vi "myRIO-1900 Quadrotor Motor MPU6050 FPGA.vi"() -> ()   [LabVIEW 2013]
uses:
  <vilib>/Platform/TimedLoop/XDataNode/timing_clust.ctl
  <vilib>/Platform/TimedLoop/XDataNode/nitl_modes.ctl
  <vilib>/Platform/TimedLoop/XDataNode/wakeup.ctl
  <vilib>/IEDriver/SPIandI2C/FPGA/Private/Initialize Port (I2C).vi
  <vilib>/IEDriver/SPIandI2C/FPGA/Private/IP Port (I2C).vi
  <vilib>/rvi/DataTransferAndStorage/Container/Common/niFpgaContainerGetUniqueNameForEmu.vi
  <vilib>/rvi/DataTransferAndStorage/Container/Common/niFpgaContainerSetEmuInfo.vi
  <vilib>/rvi/eio/common/nirviEmuReportErrorAndStop.vi
  <vilib>/rvi/Emulation/niFpgaSctlEmulationGetInTimedLoop.vi
  <vilib>/rvi/Emulation/niFpgaEmulationReportErrorSimple.vi
  <vilib>/rvi/Emulation/niFpgaGetClockAttributes.vi
  <vilib>/rvi/Emulation/niFpgaCriticalErrorInLSC.vi
  <vilib>/rvi/DataTransferAndStorage/Container/Common/niFpgaContainerExecOnDevCompGetState.vi
  <vilib>/rvi/FIFO/Fifo_Resource/nirvififoEmulationReadFpgaImpl.vi
  <vilib>/rvi/interface/RandomDataEmulation/nirviRandomDataFPGAFIFO.vi
  <vilib>/rvi/interface/RandomDataEmulation/niFpgaRandomDataHandleErrors.vi
  <vilib>/rvi/Memory/Memory_Emulation/nirvimemoryFastEmulationFpgaImpl.vi
  <instcachedir>/0/nirvimemoryFastEmulationFpgaImpl_5FBAB50466BC4C939F684F8805638BFC.lvgen/nirvimemoryFastEmulationFpgaImpl_5FBAB50466BC4C939F684F8805638BFC_005.vi
  <vilib>/rvi/Memory/Memory_Emulation/niFpgaMemoryEmulationCacheClearOnFirstRun.vi
  <vilib>/rvi/Memory/Memory_Emulation/nirvimemoryEmulationManagerCache_MakeExclusive.vi
  <vilib>/rvi/Memory/Memory_Emulation/niFpgaMemoryEmulationValidateCache.vi
  <vilib>/rvi/Memory/Memory_Emulation/nirvimemoryEmulationManagerCache_ReleaseExclusive.vi
  <vilib>/rvi/Memory/Memory_Emulation/nirvimemoryEmulationManagerCache_InsertValue.vi
  <vilib>/Utility/error.llb/Clear Errors.vi
  <vilib>/rvi/Memory/Memory_Emulation/nirvimemoryEmulationManagerCache_GetValue.vi
  <vilib>/rvi/Emulation/niFpgaProcessEmulError.vi
  <vilib>/rvi/eio/common/nirviEmuTemplateMethod_errors.vi
  <vilib>/IEDriver/SPIandI2C/FPGA/Private/Configure Port (I2C).vi
  <vilib>/IEDriver/SPIandI2C/FPGA/Private/Arm Port (I2C).vi
  <vilib>/IEDriver/SPIandI2C/FPGA/Private/Read Port (I2C).vi
  <vilib>/IEDriver/SPIandI2C/FPGA/Private/Write Port (I2C).vi
  <vilib>/rvi/FIFO/Fifo_Resource/nirvififoEmulationWriteFpgaImpl.vi
  <vilib>/rvi/Memory/Memory_Emulation/nirvimemoryEmulationManagerCache_SetValue.vi
  <vilib>/rvi/Emulation/niFpgaSctlEmulationResourceMgr.vi
  <vilib>/Platform/TimedLoop/XDataNode/XDataNode.xnode
  <vilib>/rvi/LocalResourceManager/LocalResourceManager.xnode
  <vilib>/rvi/DataTransferAndStorage/Container/XNode/niFpgaContainer.xnode
  <vilib>/rvi/FIFO/Fifo_Resource/niFpgaFifoEmulationRefIn.vi
  <vilib>/rvi/Memory/Memory_Emulation/niFpgaMemoryEmulationRefIn.vi
  <vilib>/eio/EIOMethodNode/EIOMethodNode.xnode
  <vilib>/Platform/TimedLoop/XDataNode/XDNodeRunTimeDep.lvlib
  <vilib>/IEDriver/SPIandI2C/FPGA/Library/IP SPI&I2C.lvlib
panel:
  in  "DataAva":bool
  out "GYR_Z":i16
  out "GYR_Y":i16
  out "GYR_X":i16
  out "TEMP":i16
  out "ACC_Z":i16
  out "ACC_Y":i16
  out "ACC_X":i16
  in  "SampleRate_Divider":u32=20000
  in  "WriteData":u8 format="0x%x"
  out "ReadData":u8 format="0x%x"
  in  "CMDParameters":T1
  in  "IICParameters":T2={"Address Type (7-bit)"=enum."7-bit", "IICSlaveAddress"=25, "I2C Parameters"={"Clock Divider"=0}} {"IICSlaveAddress" format="0x%x"}
  in  "ProtocolControl":T3(ring)
  in  "FeedDog":bool
  in  "CounterMAX":u32
  in  "PWM1":u16
  in  "PWM2":u16
  in  "PWM0":u16
  in  "PWM3":u16
  in  "MotorEn":bool
  in  "PWMOutputEN":bool
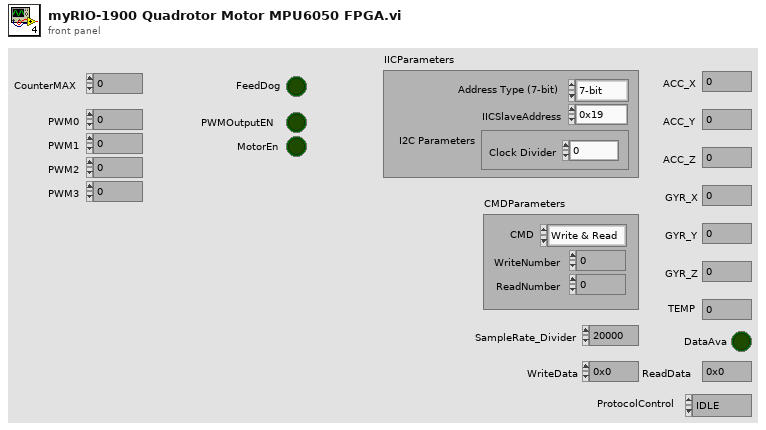
[diagram p1: front panel]
types:
  T1 = cluster{"WriteNumber":u8, "ReadNumber":u8, "CMD":enum8{"Write & Read", "Write", "Read"}}
  T2 = cluster{"Address Type (7-bit)":enum16{"7-bit", "10-bit"}, "IICSlaveAddress":u16, "I2C Parameters":cluster{"Clock Divider":u32}}
  T3 = enum8{"IDLE", "SetIDLE", "Config", "Arm", "Read", "Write", "AutoRead"}
  T4 = cluster{"MPU6050FIFO":refnum<k21>, "MPU6050FIFOAvailable":refnum<k21>}
  T5 = cluster{"PWM0":refnum<k21>, "PWM1":refnum<k21>, "PWM2":refnum<k21>, "PWM3":refnum<k21>}
  T6 = typedef "IP SPI&I2C.lvlib/Private Data (I2C).ctl" = cluster{"Arm Trigger":refnum<k21>, "API to IP Data":refnum<k21>, "IP to API Data":refnum<k21>, "Configuration Register":refnum<k21>, "Configuration Lock":refnum<k21>}
  T7 = typedef "XDNodeRunTimeDep.lvlib/timing_clust.ctl" = cluster{"Expected End [f-1]":u64, "Actual End [f-1]":u64, "Finished Late? [f-1]":bool, "Expected End [i-1]":u64, "Actual End [i-1]":u64, "Finished Late? [i-1]":bool, "Expected Start [i]":u64, "Actual Start [i]":u64, "Expected Start [f]":u64, "Actual Start [f]":u64, "Source Name":string, "Structure Name":string, "Period":i64, "Deadline":i64, "Offset":i64, "Start":i64, "Priority":i32, "Timeout":i32, "Mode":T8, "Wakeup Reason":T9, "Error":errorcluster, "Source Type":string, "Secondary Source Type":string, "Global End Time":u64, "Global Start Time":u64, "Frame Duration":u64, "Iteration Duration":u64, "Assigned CPU":i32, "I/O Scan Engine Mode":u32}
  T8 = typedef "XDNodeRunTimeDep.lvlib/nitl_modes.ctl" = enum32{"No Change", "Process missed periods, maintain original phase", "Discard missed periods, maintain original phase", "Process missed periods, ignore original phase", "Discard missed periods, ignore original phase"}
  T9 = typedef "XDNodeRunTimeDep.lvlib/wakeup.ctl" = enum32{"Normal", "Aborted", "Asynchronous wakeup", "Timing source error", "Timed loop error", "Timeout"}
  T10 = cluster{"NextState":enum8{"OutputEN", "GetInput", "Update", "CycleOver"}, "PWMCnt0":u16, "PWMCnt1":u16, "PWMCnt2":u16, "PWMCnt3":u16, "Counter":u32, "WatchDog":u32, "TimeOut?":bool, "CounterMAX":u32}
  T11 = enum8{"OutputEN", "GetInput", "Update", "CycleOver"}
  T12 = cluster{"NextState":enum16{"Configure", "WriteAddr", "Arm", "Read", "Wait", "Stop"}, "ReadCount":u8, "WaitCounter":u32}
  T13 = enum16{"Configure", "WriteAddr", "Arm", "Read", "Wait", "Stop"}
  T14 = cluster{"NextState":enum8{"IDLE", "ReadData", "Update"}, "ReadCounter":u8, "HighByte":u8}
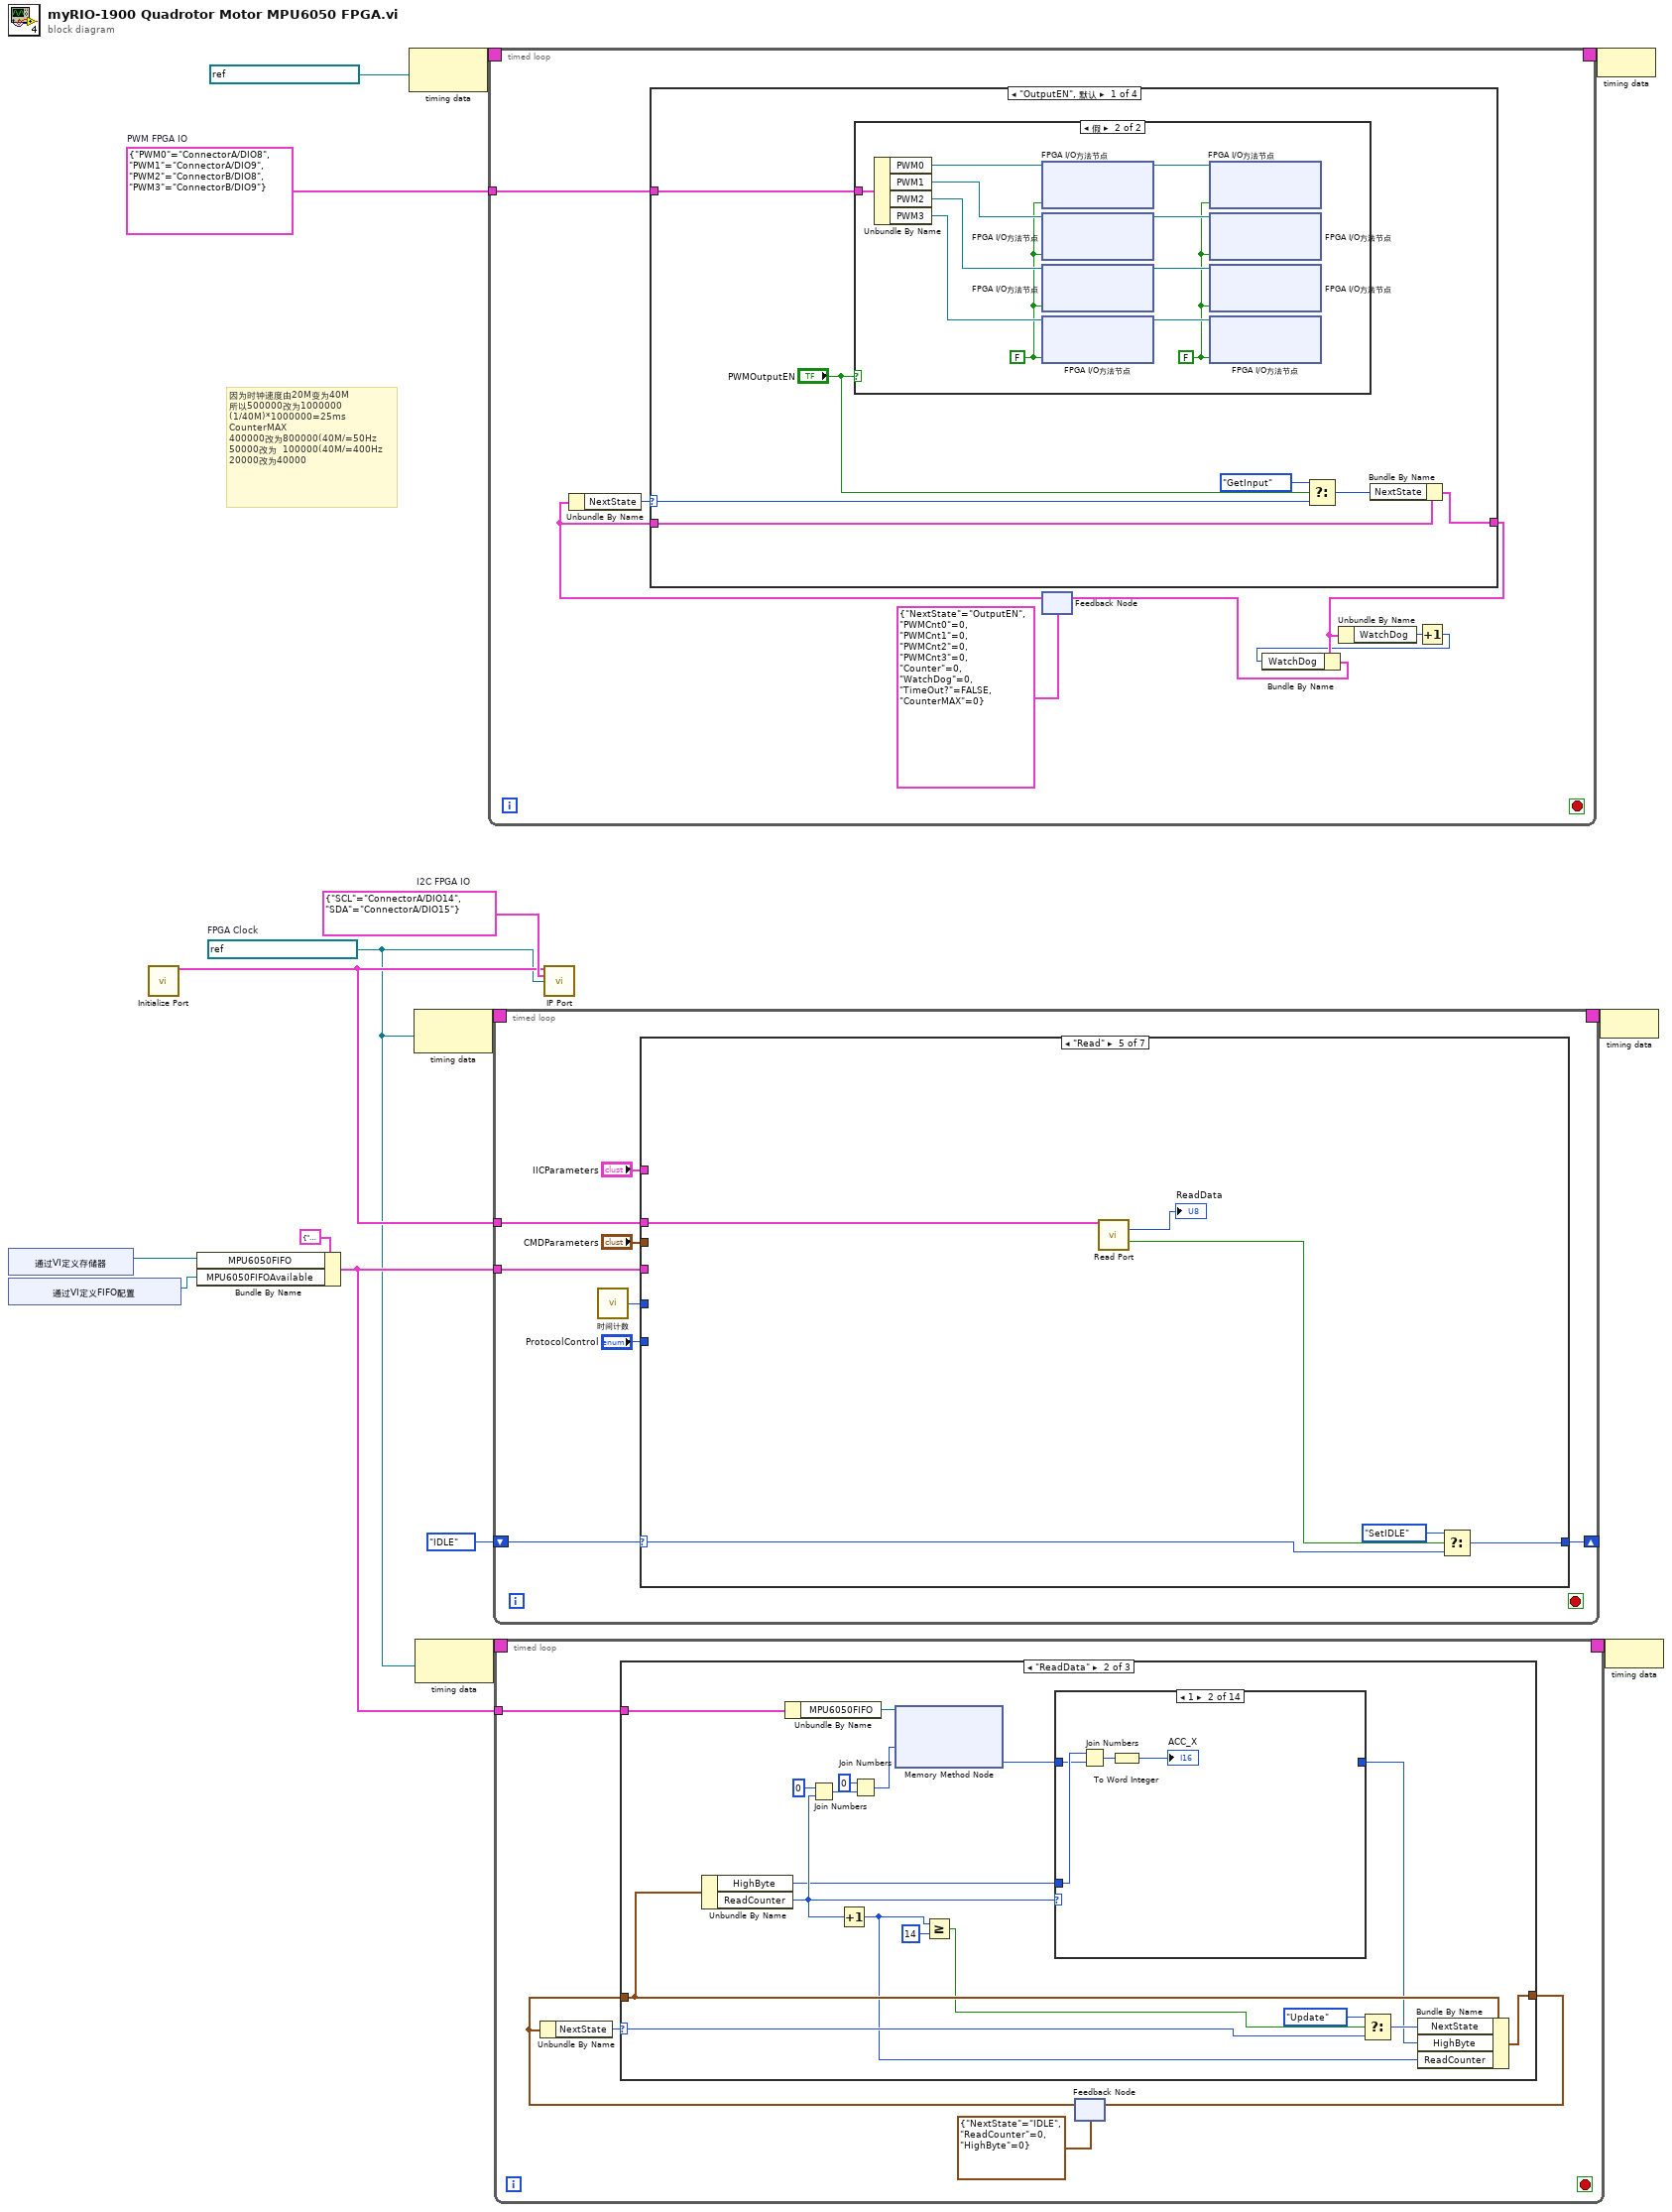
[diagram p0: block diagram]
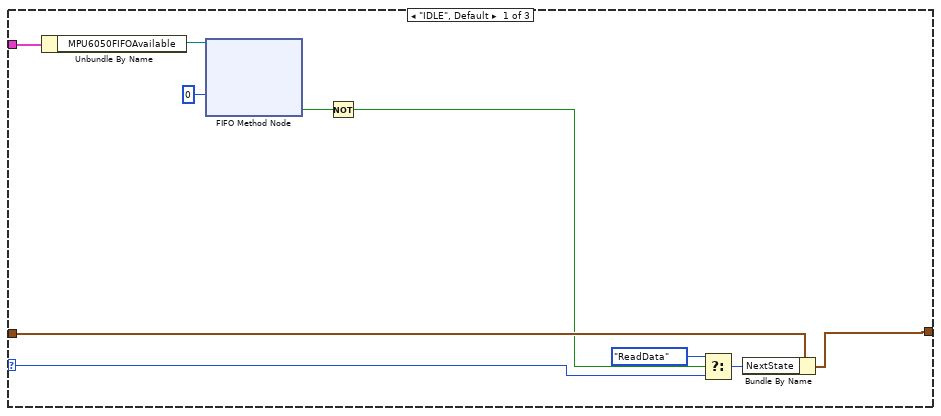
[diagram p2: hidden frame]
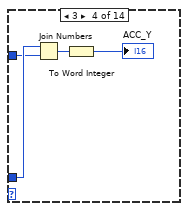
[diagram p5: hidden frame]
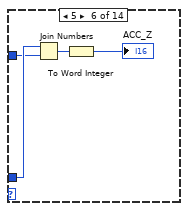
[diagram p7: hidden frame]
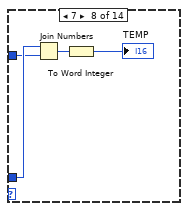
[diagram p9: hidden frame]
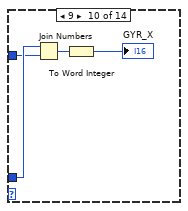
[diagram p11: hidden frame]
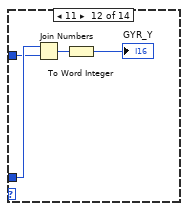
[diagram p13: hidden frame]
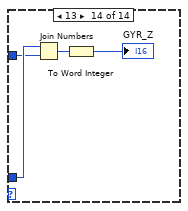
[diagram p15: hidden frame]
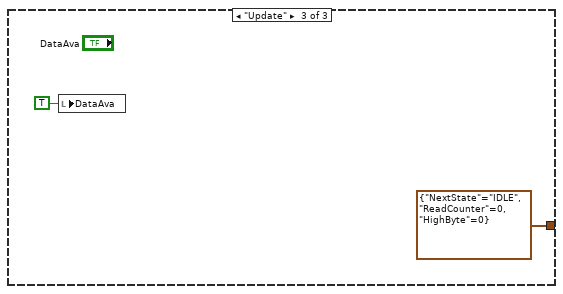
[diagram p16: hidden frame]
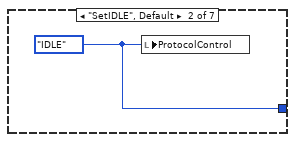
[diagram p18: hidden frame]
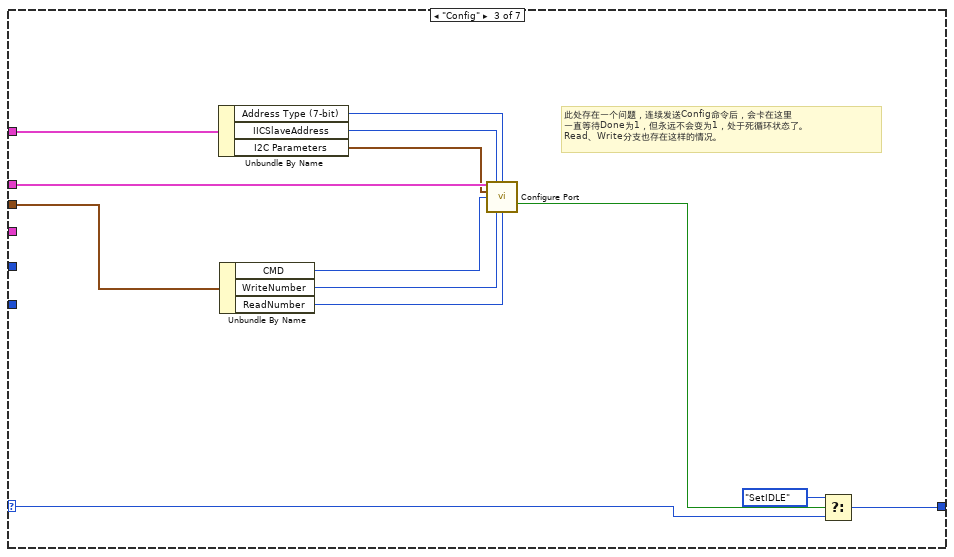
[diagram p19: hidden frame]
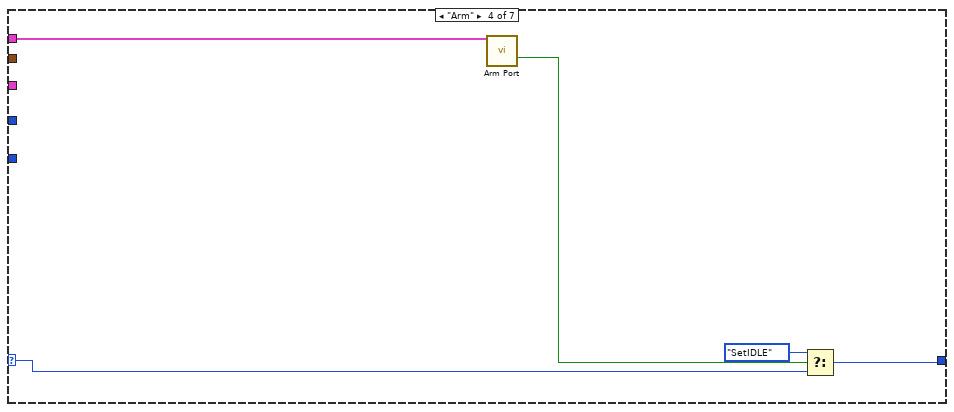
[diagram p20: hidden frame]
diagram:
  w1 = refnum<k21> "40 MHz Onboard Clock"  # FPGA Clock
  w8 = cluster{"SCL":refnum<k21>, "SDA":refnum<k21>} {"SCL"="ConnectorA/DIO14", "SDA"="ConnectorA/DIO15"}  # I2C FPGA IO
  w14 = T5 {"PWM0"="ConnectorA/DIO8", "PWM1"="ConnectorA/DIO9", "PWM2"="ConnectorB/DIO8", "PWM3"="ConnectorB/DIO9"}  # PWM FPGA IO
  # "因为时钟速度由20M变为40M\n所以500000改为1000000\n(1/40M)*1000000=25ms\nCounterMAX\n400000改为800000(40M/=50Hz\n50000改为  100000(40M/=400Hz\n20000改为40000"
  n1 = xnode "通过VI定义存储器"() -> ("存储器输出"=w4:refnum<k21>)
  n2 = xnode "通过VI定义FIFO配置"() -> ("FIFO输出"=w3:refnum<k21>)
  n3 = call-poly <vilib>:"Initialize Port.vi"() -> ("Private Data Out"=w7:T6)  [unwired: 14 in, 1 out]
  n4 = Bundle By Name(cluster=T4 {"MPU6050FIFO"="", "MPU6050FIFOAvailable"=""}, "MPU6050FIFO"=w4, "MPU6050FIFOAvailable"=w3) -> (w2:T4)
  n5 = node-c288(refnum<k21> "40 MHz Onboard Clock" ("源名称")) -> (w16:T7)
  n6 = node-c288(w1) -> (w12:T7)
  n7 = node-c288(w1) -> (w10:T7)
  n8 = timed-loop {
    timing: w16 -> [_]
    timing-out: [_] -> w15
    tunnel: w14 -> [w21]
    stop <- _ stop-if-true
    n9 = feedback #1(T10 {"NextState"=enum."OutputEN", "PWMCnt0"=0, "PWMCnt1"=0, "PWMCnt2"=0, "PWMCnt3"=0, "Counter"=0, "WatchDog"=0, "TimeOut?"=FALSE, "CounterMAX"=0}) -> (w23:T10)
    n10 = Unbundle By Name(w23) -> ("NextState"=w22:T11)
    n11 = case shown="\"OutputEN\", 默认" w22 {
      selector: w22 -> [w27 _ _ _]
      tunnel: w23 -> [w30 w74 w109 w130]
      tunnel: [w29 w75 w108 w129] -> w20
      tunnel: w21 -> [w31 _ w122 _]
      frame "OutputEN", Default {
        n12 = case shown="假" "PWMOutputEN" {
          tunnel: w31 -> [w42 w53]
          frame True {
            w32 = FALSE ("启用")
            w37 = TRUE ("启用")
            n13 = Unbundle By Name(w42) -> ("PWM0"=w41:refnum<k21>, "PWM1"=w38:refnum<k21>, "PWM2"=w40:refnum<k21>, "PWM3"=w39:refnum<k21>)
            n14 = xnode "FPGA I/O方法节点"("FPGA I/O In"=w41, "启用"=w37) -> ("FPGA I/O Out"=w36:refnum<k21>)
            n15 = xnode "FPGA I/O方法节点"("FPGA I/O In"=w38, "启用"=w37) -> ("FPGA I/O Out"=w35:refnum<k21>)
            n16 = xnode "FPGA I/O方法节点"("FPGA I/O In"=w40, "启用"=w37) -> ("FPGA I/O Out"=w34:refnum<k21>)
            n17 = xnode "FPGA I/O方法节点"("FPGA I/O In"=w39, "启用"=w37) -> ("FPGA I/O Out"=w33:refnum<k21>)
            n18 = xnode "FPGA I/O方法节点"("FPGA I/O In"=w36, "数据"=w32) -> ()  [unwired: 1 out]
            n19 = xnode "FPGA I/O方法节点"("FPGA I/O In"=w35, "数据"=w32) -> ()  [unwired: 1 out]
            n20 = xnode "FPGA I/O方法节点"("FPGA I/O In"=w34, "数据"=w32) -> ()  [unwired: 1 out]
            n21 = xnode "FPGA I/O方法节点"("FPGA I/O In"=w33, "数据"=w32) -> ()  [unwired: 1 out]
          }
          frame False {
            w43 = FALSE ("启用")
            w48 = FALSE ("启用")
            n22 = Unbundle By Name(w53) -> ("PWM0"=w52:refnum<k21>, "PWM1"=w49:refnum<k21>, "PWM2"=w51:refnum<k21>, "PWM3"=w50:refnum<k21>)
            n23 = xnode "FPGA I/O方法节点"("FPGA I/O In"=w52, "启用"=w48) -> ("FPGA I/O Out"=w47:refnum<k21>)
            n24 = xnode "FPGA I/O方法节点"("FPGA I/O In"=w49, "启用"=w48) -> ("FPGA I/O Out"=w46:refnum<k21>)
            n25 = xnode "FPGA I/O方法节点"("FPGA I/O In"=w51, "启用"=w48) -> ("FPGA I/O Out"=w45:refnum<k21>)
            n26 = xnode "FPGA I/O方法节点"("FPGA I/O In"=w50, "启用"=w48) -> ("FPGA I/O Out"=w44:refnum<k21>)
            n27 = xnode "FPGA I/O方法节点"("FPGA I/O In"=w47, "数据"=w43) -> ()  [unwired: 1 out]
            n28 = xnode "FPGA I/O方法节点"("FPGA I/O In"=w46, "数据"=w43) -> ()  [unwired: 1 out]
            n29 = xnode "FPGA I/O方法节点"("FPGA I/O In"=w45, "数据"=w43) -> ()  [unwired: 1 out]
            n30 = xnode "FPGA I/O方法节点"("FPGA I/O In"=w44, "数据"=w43) -> ()  [unwired: 1 out]
          }
        }
        n31 = Select(t=T11."GetInput", s="PWMOutputEN", f=w27) -> (s? t:f=w26:T11)
        n32 = Bundle By Name(cluster=w30, "NextState"=w26) -> (w29:T10)
      }
      frame "GetInput" {
        # "25ms"
        n33 = Unbundle By Name(w74) -> ("CounterMAX"=w58:u32, "TimeOut?"=w71:bool, "WatchDog"=w69:u32)
        n34 = Greater Or Equal?(x=w69, y=u32 1000000) -> (x >= y?=w72:bool)
        n35 = Or(x=w71, y=w72) -> (x .or. y?=w55:bool)
        n36 = Select(t=u32 0, s="FeedDog", f=w69) -> (s? t:f=w70:u32)
        n37 = Not(x="MotorEn") -> (.not. x?=w54:bool)
        n38 = Not(x="FeedDog") -> (.not. x?=w66:bool)
        n39 = And(x=w55, y=w66) -> (x .and. y?=w59:bool)
        n40 = Or(x=w54, y=w55) -> (x .or. y?=w56:bool)
        n41 = case shown="假" w56 {
          tunnel: [w90 u16 40000 ("PWM0")] -> w65
          tunnel: [w89 u16 40000 ("PWM1")] -> w64
          tunnel: [w88 u16 40000 ("PWM2")] -> w63
          tunnel: [w87 u16 40000 ("PWM3")] -> w62
          tunnel: [w92 w97] -> w61
          tunnel: w58 -> [_ w97]
          frame False {
            w82 = u16 0 ("PWM1")
            w81 = u16 40000 ("PWM1")
            w91 = u16 40000
            n42 = In Range and Coerce(upper limit=w81, x="PWM0", lower limit=w82) -> (coerced(x)=w80:u16)  [unwired: 1 out]
            n43 = In Range and Coerce(upper limit=w81, x="PWM1", lower limit=w82) -> (coerced(x)=w79:u16)  [unwired: 1 out]
            n44 = In Range and Coerce(upper limit=w81, x="PWM2", lower limit=w82) -> (coerced(x)=w78:u16)  [unwired: 1 out]
            n45 = In Range and Coerce(upper limit=w81, x="PWM3", lower limit=w82) -> (coerced(x)=w77:u16)  [unwired: 1 out]
            n46 = In Range and Coerce(upper limit=u32 800000 ("上限"), x="CounterMAX", lower limit=u32 100000 ("下限")) -> (coerced(x)=w92:u32)  [unwired: 1 out]
            n47 = Add(x=w80, y=w91) -> (x+y=w90:u16)
            n48 = Add(x=w79, y=w91) -> (x+y=w89:u16)
            n49 = Add(x=w78, y=w91) -> (x+y=w88:u16)
            n50 = Add(x=w77, y=w91) -> (x+y=w87:u16)
          }
          frame True {
          }
        }
        n51 = flat-sequence {
          tunnel: w59 -> [_]
          frame #0 {
            n52 = local write "FeedDog"(FALSE ("FeedDog")) -> ()
          }
        }
        n53 = Bundle By Name(cluster=w74, "PWMCnt0"=w65, "PWMCnt1"=w64, "PWMCnt2"=w63, "PWMCnt3"=w62, "CounterMAX"=w61, "WatchDog"=w70, "TimeOut?"=w59, "NextState"=T11."Update") -> (w75:T10)
      }
      frame "Update" {
        n54 = Unbundle By Name(w109) -> ("Counter"=w113:u32, "PWMCnt0"=w126:u16, "PWMCnt1"=w125:u16, "PWMCnt2"=w124:u16, "PWMCnt3"=w123:u16, "CounterMAX"=w112:u32, "NextState"=w110:T11)
        n55 = To Unsigned Long Integer(number=w126) -> (unsigned 32bit integer=w104:u32)
        n56 = To Unsigned Long Integer(number=w125) -> (unsigned 32bit integer=w103:u32)
        n57 = To Unsigned Long Integer(number=w124) -> (unsigned 32bit integer=w102:u32)
        n58 = To Unsigned Long Integer(number=w123) -> (unsigned 32bit integer=w101:u32)
        n59 = Less?(x=w113, y=w104) -> (x < y?=w117:bool)
        n60 = Less?(x=w113, y=w103) -> (x < y?=w116:bool)
        n61 = Unbundle By Name(w122) -> ("PWM0"=w121:refnum<k21>, "PWM1"=w120:refnum<k21>, "PWM2"=w119:refnum<k21>, "PWM3"=w118:refnum<k21>)
        n62 = Less?(x=w113, y=w102) -> (x < y?=w115:bool)
        n63 = Less?(x=w113, y=w101) -> (x < y?=w114:bool)
        n64 = Increment(x=w113) -> (x+1=w105:u32)
        n65 = Greater?(x=w105, y=w112) -> (0:w111:bool)
        n66 = xnode "FPGA I/O方法节点"("FPGA I/O In"=w121, "数据"=w117) -> ()  [unwired: 1 out]
        n67 = xnode "FPGA I/O方法节点"("FPGA I/O In"=w120, "数据"=w116) -> ()  [unwired: 1 out]
        n68 = xnode "FPGA I/O方法节点"("FPGA I/O In"=w119, "数据"=w115) -> ()  [unwired: 1 out]
        n69 = xnode "FPGA I/O方法节点"("FPGA I/O In"=w118, "数据"=w114) -> ()  [unwired: 1 out]
        n70 = Select(t=T11."CycleOver", s=w111, f=w110) -> (s? t:f=w107:T11)
        n71 = Bundle By Name(cluster=w109, "Counter"=w105, "NextState"=w107) -> (w108:T10)
      }
      frame "CycleOver" {
        n72 = Bundle By Name(cluster=w130, "Counter"=u32 0, "NextState"=T11."OutputEN") -> (w129:T10)
      }
    }
    n73 = Unbundle By Name(w20) -> ("WatchDog"=w19:u32)
    n74 = Increment(x=w19) -> (x+1=w18:u32)
    n75 = Bundle By Name(cluster=w20, "WatchDog"=w18) -> (w17:T10)
    n76 = feedback-in #1(w17) -> ()
  }
  n77 = timed-loop {
    tunnel: w7 -> [w138]
    shift-right: [w135] -> _
    shift-left: T3."IDLE" ("ProtocolControl") -> [w140]
    timing: w12 -> [_]
    timing-out: [_] -> w11
    tunnel: w2 -> [w133]
    stop <- _ stop-if-true
    n78 = call "时间计数"() -> ("Tick Count(Ticks)"=w134:u32)
    n79 = case shown="\"Read\"" w140 {
      selector: w140 -> [_ _ w155 w158 w165 w170 w183]
      tunnel: "CMDParameters" -> [_ _ w148 _ _ _ _]
      tunnel: w138 -> [_ _ w154 w160 w166 w172 w179]
      tunnel: "IICParameters" -> [_ _ w152 _ _ _ w178]
      tunnel: "ProtocolControl" -> [w141 _ _ _ _ _ w177]
      tunnel: [w141 w142 w144 w157 w162 w168 w184] -> w135
      tunnel: w134 -> [_ _ _ _ _ _ w175]
      tunnel: w133 -> [_ _ _ _ _ _ w174]
      frame "IDLE" {
      }
      frame "SetIDLE", Default {
        w142 = T3."IDLE" ("ProtocolControl")
        n80 = local write "ProtocolControl"(w142) -> ()
      }
      frame "Config" {
        # "此处存在一个问题，连续发送Config命令后，会卡在这里\n一直等待Done为1，但永远不会变为1，处于死循环状态了。\nRead、Write分支也存在这样的情况。"
        n81 = Unbundle By Name(w152) -> ("Address Type (7-bit)"=w151:enum16{"7-bit", "10-bit"}, "IICSlaveAddress"=w150:u16, "I2C Parameters"=w149:cluster{"Clock Divider":u32})
        n82 = Unbundle By Name(w148) -> ("CMD"=w147:enum8{"Write & Read", "Write", "Read"}, "WriteNumber"=w146:u8, "ReadNumber"=w145:u8)
        n83 = call-poly <vilib>:"Configure Port.vi"("Private Data In"=w154, "Address"=w150, "Address Type (7-bit)"=w151, "I2C Parameters"=w149, "Command (Write & Read)"=w147, "Number of Bytes to Write"=w146, "Number of Bytes to Read"=w145) -> ("Done"=w153:bool)  [unwired: 6 in, 2 out]
        n84 = Select(t=T3."SetIDLE", s=w153, f=w155) -> (s? t:f=w144:T3)
      }
      frame "Arm" {
        n85 = call-poly <vilib>:"Arm Port.vi"("Private Data In"=w160) -> ("Done"=w159:bool)  [unwired: 12 in, 2 out]
        n86 = Select(t=T3."SetIDLE", s=w159, f=w158) -> (s? t:f=w157:T3)
      }
      frame "Read" {
        n87 = call-poly <vilib>:"Read Port.vi"("Private Data In"=w166) -> ("Data Out"=→"ReadData":u8, "Output Valid"=w164:bool)  [unwired: 11 in, 2 out]
        n88 = Select(t=T3."SetIDLE", s=w164, f=w165) -> (s? t:f=w162:T3)
      }
      frame "Write" {
        n89 = call-poly <vilib>:"Write Port.vi"("Private Data In"=w172, "Data In"="WriteData") -> ("Done"=w169:bool)  [unwired: 11 in, 2 out]
        n90 = Select(t=T3."SetIDLE", s=w169, f=w170) -> (s? t:f=w168:T3)
      }
      frame "AutoRead" {
        n91 = feedback #2(T12 {"NextState"=enum."Configure", "ReadCount"=0, "WaitCounter"=0}) -> (w181:T12)
        n92 = Unbundle By Name(w181) -> ("NextState"=w173:T13)
        n93 = case shown="\"Read\"" w173 {
          selector: w173 -> [w190 w204 w213 w224 w249 _]
          tunnel: w181 -> [w192 w203 w211 w222 w251 _]
          tunnel: [w191 w202 w212 w223 w250 T12 {"NextState"=enum."Configure", "ReadCount"=0, "WaitCounter"=0}] -> w180
          tunnel: w179 -> [w200 w208 w210 w227 _ _]
          tunnel: w178 -> [w199 _ _ _ _ _]
          tunnel: w177 -> [_ _ _ _ _ w257]
          tunnel: [_ _ _ _ _ w255] -> w176
          tunnel: w175 -> [w186 _ _ _ w245 _]
          tunnel: w174 -> [_ _ _ w217 _ _]
          frame "Configure", Default {
            w195 = u8 0 items=["Write & Read", "Write", "Read"] ("Command (Write & Read)")
            # "NO Done"
            n94 = Unbundle By Name(w199) -> ("Address Type (7-bit)"=w198:enum16{"7-bit", "10-bit"}, "IICSlaveAddress"=w197:u16, "I2C Parameters"=w196:cluster{"Clock Divider":u32})
            n95 = call-poly <vilib>:"Configure Port.vi"("Private Data In"=w200, "Address"=w197, "Address Type (7-bit)"=w198, "I2C Parameters"=w196, "Command (Write & Read)"=w195, "Number of Bytes to Write"=u16 1, "Number of Bytes to Read"=u16 14) -> ("Done"=w188:bool)  [unwired: 6 in, 2 out]
            n96 = Select(t=T13."WriteAddr", s=w188, f=w190) -> (s? t:f=w189:T13)
            n97 = Bundle By Name(cluster=w192, "NextState"=w189, "WaitCounter"=w186) -> (w191:T12)
          }
          frame "WriteAddr" {
            n98 = call-poly <vilib>:"Write Port.vi"("Private Data In"=w208, "Data In"=u8 59) -> ("Done"=w201:bool)  [unwired: 11 in, 2 out]
            n99 = Select(t=T13."Arm", s=w201, f=w204) -> (s? t:f=w206:T13)
            n100 = Bundle By Name(cluster=w203, "NextState"=w206) -> (w202:T12)
          }
          frame "Arm" {
            n101 = call-poly <vilib>:"Arm Port.vi"("Private Data In"=w210) -> ("Done"=w209:bool)  [unwired: 12 in, 2 out]
            n102 = Select(t=T13."Read", s=w209, f=w213) -> (s? t:f=w215:T13)
            n103 = Bundle By Name(cluster=w211, "NextState"=w215) -> (w212:T12)
          }
          frame "Read" {
            n104 = Unbundle By Name(w222) -> ("ReadCount"=w226:u8)
            n105 = call-poly <vilib>:"Read Port.vi"("Private Data In"=w227) -> ("Data Out"=w225:u8, "Output Valid"=w216:bool)  [unwired: 11 in, 2 out]
            n106 = case shown="假" w216 {
              tunnel: w226 -> [w231 w240]
              tunnel: w225 -> [_ w237]
              tunnel: [w231 w244] -> w220
              tunnel: w217 -> [w232 w239]
              frame False {
                n107 = Unbundle By Name(w232) -> ("MPU6050FIFOAvailable"=w229:refnum<k21>)
                n108 = Less Or Equal?(x=u8 13, y=w231) -> (x <= y?=w228:bool)
                n109 = case shown="真" w228 {
                  tunnel: w229 -> [_ w235]
                  frame False {
                  }
                  frame True {
                    n110 = xnode ("FIFO Method Node")("元素"=TRUE, "超时"=0, "FIFO输入"=w235) -> ()  [unwired: 2 out]
                  }
                }
              }
              frame True {
                n111 = Unbundle By Name(w239) -> ("MPU6050FIFO"=w238:refnum<k21>)
                n112 = Join Numbers(hi=u8 0, lo=w240) -> ((hi.lo)=w243:u16)
                n113 = Join Numbers(hi=u16 0, lo=w243) -> ((hi.lo)=w236:u32)
                n114 = Increment(x=w240) -> (x+1=w244:u8)
                n115 = xnode ("Memory Method Node")("地址"=w236, "数据"=w237, "存储器输入"=w238) -> ()  [unwired: 1 out]
              }
            }
            n116 = Not(x=w216) -> (.not. x?=w219:bool)
            n117 = Select(t=T13."Wait", s=w219, f=w224) -> (s? t:f=w221:T13)
            n118 = Bundle By Name(cluster=w222, "ReadCount"=w220, "NextState"=w221) -> (w223:T12)
          }
          frame "Wait" {
            n119 = Unbundle By Name(w251) -> ("WaitCounter"=w254:u32)
            n120 = Subtract(x=w245, y=w254) -> (x-y=w253:u32)
            n121 = Less?(x="SampleRate_Divider", y=w253) -> (x < y?=w247:bool)
            n122 = Select(t=T13."Stop", s=w247, f=w249) -> (s? t:f=w248:T13)
            n123 = Bundle By Name(cluster=w251, "NextState"=w248) -> (w250:T12)
          }
          frame "Stop" {
            # "Done"
            n124 = Equal?(x=T3."SetIDLE", y=w257) -> (x = y?=w255:bool)
          }
        }
        n125 = feedback-in #2(w180) -> ()
        n126 = Select(t=T3."SetIDLE", s=w176, f=w183) -> (s? t:f=w184:T3)
      }
    }
  }
  n127 = timed-loop {
    tunnel: w2 -> [w262]
    timing: w10 -> [_]
    timing-out: [_] -> w9
    stop <- _ stop-if-true
    n128 = feedback #3(T14 {"NextState"=enum."IDLE", "ReadCounter"=0, "HighByte"=0}) -> (w264:T14)
    n129 = Unbundle By Name(w264) -> ("NextState"=w263:enum8{"IDLE", "ReadData", "Update"})
    n130 = case shown="\"ReadData\"" w263 {
      selector: w263 -> [w270 w284 _]
      tunnel: w264 -> [w272 w286 _]
      tunnel: w262 -> [w275 w293 _]
      tunnel: [w271 w285 T14 {"NextState"=enum."IDLE", "ReadCounter"=0, "HighByte"=0}] -> w261
      frame "IDLE", Default {
        n131 = Unbundle By Name(w275) -> ("MPU6050FIFOAvailable"=w274:refnum<k21>)
        n132 = xnode ("FIFO Method Node")("超时"=0, "FIFO输入"=w274) -> ("超时？"=w268:bool)  [unwired: 2 out]
        n133 = Not(x=w268) -> (.not. x?=w267:bool)
        n134 = Select(t=enum8{"IDLE", "ReadData", "Update"}."ReadData", s=w267, f=w270) -> (s? t:f=w269:enum8{"IDLE", "ReadData", "Update"})
        n135 = Bundle By Name(cluster=w272, "NextState"=w269) -> (w271:T14)
      }
      frame "ReadData" {
        n136 = Unbundle By Name(w286) -> ("HighByte"=w277:u8, "ReadCounter"=w280:u8)
        n137 = Unbundle By Name(w293) -> ("MPU6050FIFO"=w292:refnum<k21>)
        n138 = Join Numbers(hi=u8 0, lo=w280) -> ((hi.lo)=w291:u16)
        n139 = Increment(x=w280) -> (x+1=w276:u8)
        n140 = Join Numbers(hi=u16 0, lo=w291) -> ((hi.lo)=w288:u32)
        n141 = xnode ("Memory Method Node")("地址"=w288, "存储器输入"=w292) -> ("数据"=w279:u8)  [unwired: 1 out]
        n142 = Greater Or Equal?(x=w276, y=u8 14) -> (x >= y?=w282:bool)
        n143 = case shown="1" w280 {
          tunnel: w279 -> [w294 w297 w299 w302 w304 w307 w309 w312 w314 w317 w319 w322 w324 w327]
          tunnel: [w294 _ w299 _ w304 _ w309 _ w314 _ w319 _ w324 _] -> w278
          tunnel: w277 -> [_ w298 _ w303 _ w308 _ w313 _ w318 _ w323 _ w328]
          frame 0, Default {
          }
          frame 1 {
            n144 = Join Numbers(hi=w298, lo=w297) -> ((hi.lo)=w296:u16)
            n145 = To Word Integer(number=w296) -> (16bit integer=→"ACC_X":i16)
          }
          frame 2 {
          }
          frame 3 {
            n146 = Join Numbers(hi=w303, lo=w302) -> ((hi.lo)=w301:u16)
            n147 = To Word Integer(number=w301) -> (16bit integer=→"ACC_Y":i16)
          }
          frame 4 {
          }
          frame 5 {
            n148 = Join Numbers(hi=w308, lo=w307) -> ((hi.lo)=w306:u16)
            n149 = To Word Integer(number=w306) -> (16bit integer=→"ACC_Z":i16)
          }
          frame 6 {
          }
          frame 7 {
            n150 = Join Numbers(hi=w313, lo=w312) -> ((hi.lo)=w311:u16)
            n151 = To Word Integer(number=w311) -> (16bit integer=→"TEMP":i16)
          }
          frame 8 {
          }
          frame 9 {
            n152 = Join Numbers(hi=w318, lo=w317) -> ((hi.lo)=w316:u16)
            n153 = To Word Integer(number=w316) -> (16bit integer=→"GYR_X":i16)
          }
          frame 10 {
          }
          frame 11 {
            n154 = Join Numbers(hi=w323, lo=w322) -> ((hi.lo)=w321:u16)
            n155 = To Word Integer(number=w321) -> (16bit integer=→"GYR_Y":i16)
          }
          frame 12 {
          }
          frame 13 {
            n156 = Join Numbers(hi=w328, lo=w327) -> ((hi.lo)=w326:u16)
            n157 = To Word Integer(number=w326) -> (16bit integer=→"GYR_Z":i16)
          }
        }
        n158 = Select(t=enum8{"IDLE", "ReadData", "Update"}."Update", s=w282, f=w284) -> (s? t:f=w283:enum8{"IDLE", "ReadData", "Update"})
        n159 = Bundle By Name(cluster=w286, "NextState"=w283, "HighByte"=w278, "ReadCounter"=w276) -> (w285:T14)
      }
      frame "Update" {
        n160 = local write "DataAva"(TRUE ("DataAva")) -> ()
      }
    }
    n161 = feedback-in #3(w261) -> ()
  }
  n162 = call-poly <vilib>:"IP Port.vi"("Private Data In"=w7, "I2C FPGA IO"=w8, "FPGA Clock"=w1) -> ()  [unwired: 13 in]
  n163 = node-c288(w15) -> ()
  n164 = node-c288(w11) -> ()
  n165 = node-c288(w9) -> ()
